vi "Add.vi"(8 "error in (no error)":errorcluster, 10 "Runnable":refnum<class "Runnable.lvclass">, 11 "LUnit Test Suite In":refnum<class "LUnit Test Suite.lvclass">) -> (0 "error out":errorcluster, 3 "LUnit Test Suite Out":refnum<class "LUnit Test Suite.lvclass">)   [LabVIEW 2020, in "LUnit Test Suite.lvclass"]
doc: "Add a test method to the test suite. Order of tests will be alphabetic regardless of the order they are added to suite."
uses:
  LUnit Test Suite.lvclass
  Runnable.lvclass
  LUnit Test Suite.lvclass/LUnit Test Suite.ctl
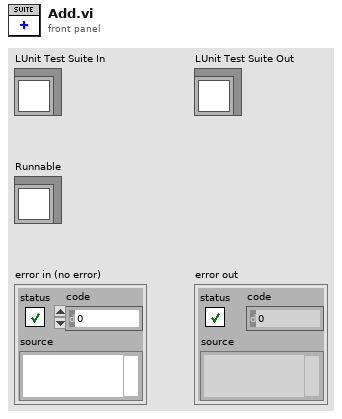
[diagram p1: front panel]
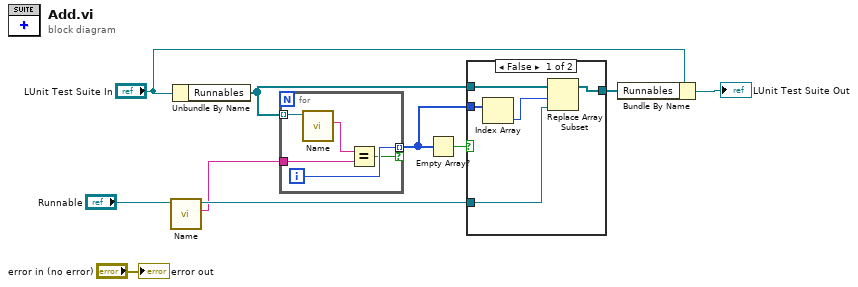
[diagram p0: block diagram]
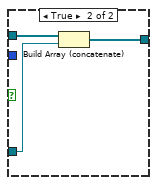
[diagram p2: hidden frame]
diagram:
  n1 = call-dynamic "Name.vi"("Runnable in"="Runnable") -> ("Name"=w4:string, "Runnable out"=w5:refnum<class "Runnable.lvclass">)  [unwired: 8 in, 1 out]
  n2 = Unbundle By Name("LUnit Test Suite In") -> ("Runnables"=w2:refnum<class "Runnable.lvclass">[])
  n3 = for {
    tunnel: w2 -> [w15] mode=indexing
    tunnel: w4 -> [w13]
    tunnel: [w12] -> w3 mode=indexing if=w11
    i -> [w12]
    n4 = call-dynamic "Name.vi"("Runnable in"=w15) -> ("Name"=w14:string)  [unwired: 8 in, 2 out]
    n5 = Equal?(x=w14, y=w13) -> (x = y?=w11:bool)
  }
  n6 = Empty Array?(array=w3) -> (empty?=w1:bool)
  n7 = case shown="False" w1 {
    tunnel: [w19 w23] -> w7
    tunnel: w5 -> [w16 w22]
    tunnel: w2 -> [w20 w21]
    tunnel: w3 -> [w18 _]
    frame False {
      n8 = Index Array(array=w18) -> (element=w17:i32)  [unwired: 1 in]
      n9 = Replace Array Subset(array=w20, new element=w16, index=w17) -> (w19:refnum<class "Runnable.lvclass">[])
    }
    frame True {
      n10 = Build Array (concatenate)(w21, w22) -> (w23:refnum<class "Runnable.lvclass">[])
    }
  }
  n11 = Bundle By Name(cluster="LUnit Test Suite In", "Runnables"=w7) -> (→"LUnit Test Suite Out":refnum<class "LUnit Test Suite.lvclass">)
  "error out" <- "error in (no error)"
